vi "Generator.vi"(9 "Distance":dbl, 10 "Velocity Max":dbl, 11 "Acceleration Max":dbl) -> (2 "Velocity values":dbl[](array[numeric]), 3 "Timestamp":dbl[](array[numeric]) format="%.2f")   [LabVIEW 2023]
panel:
  out "area":sgl
  out "Time":sgl
  out "XY Graph":cluster{dbl[], dbl[]}(graph)
  out "Slope Change Point (seconds)":dbl
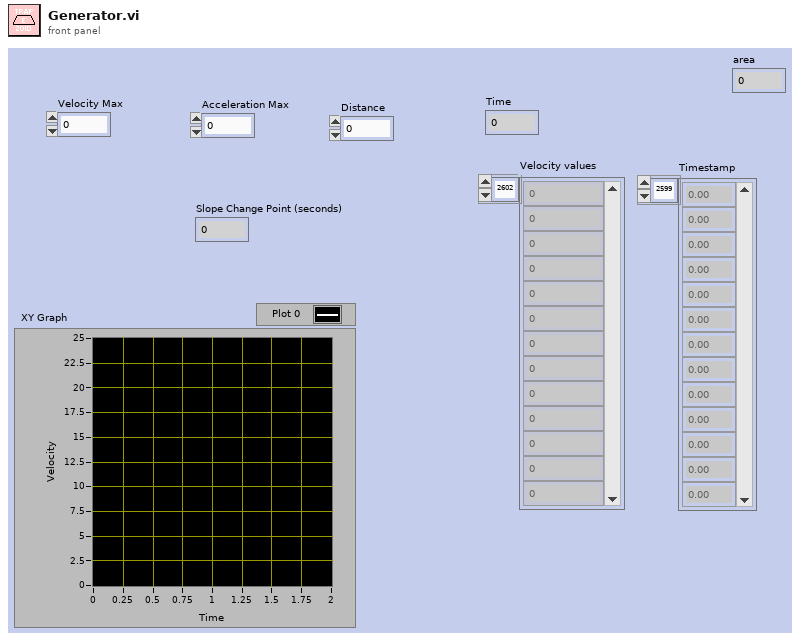
[diagram p1: front panel]
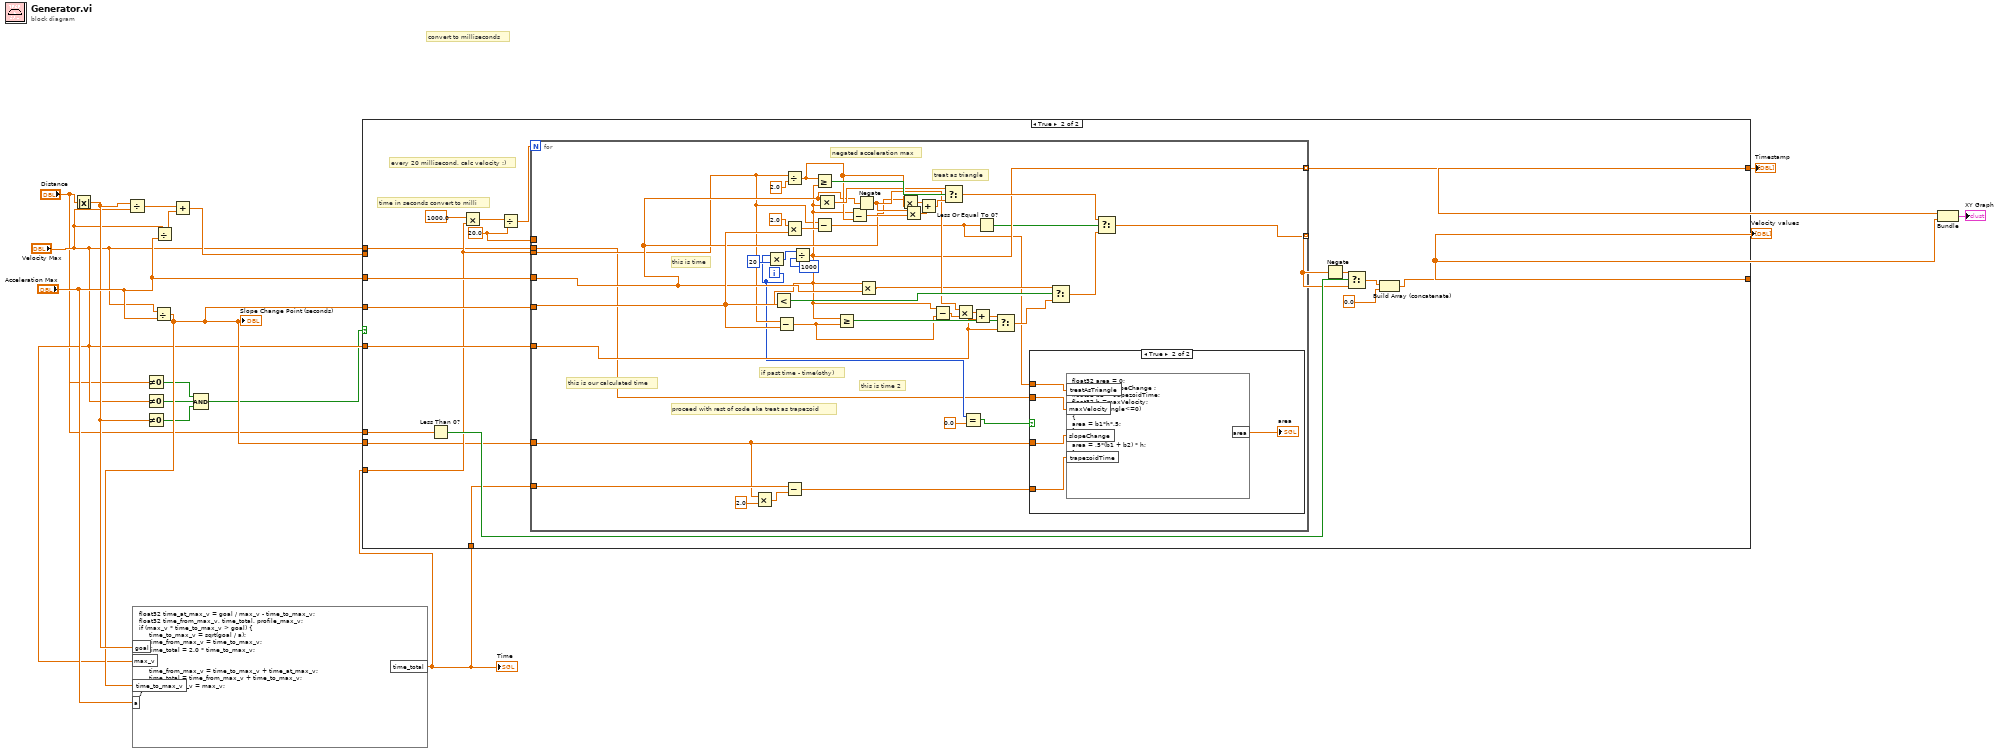
[diagram p0: block diagram]
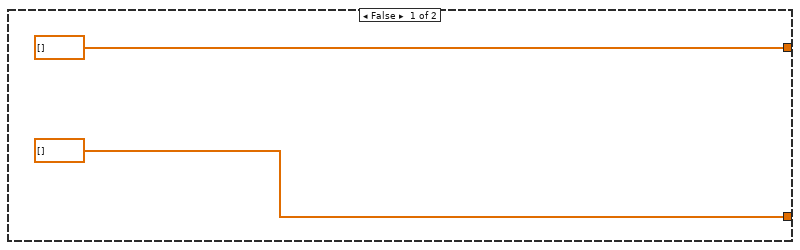
[diagram p2: hidden frame]
diagram:
  # "convert to milliseconds"
  n1 = Absolute Value(x="Distance") -> (abs(x)=w9:dbl)
  n2 = Divide(x=w9, y="Velocity Max") -> (x/y=w13:dbl)
  n3 = Not Equal To 0?(x="Distance") -> (x != 0?=w3:bool)
  n4 = Not Equal To 0?(x="Velocity Max") -> (x != 0?=w5:bool)
  n5 = Not Equal To 0?(x=w9) -> (x != 0?=w6:bool)
  n6 = Divide(x="Velocity Max", y="Acceleration Max") -> (x/y=w8:dbl)
  "Slope Change Point (seconds)" <- w8
  n7 = formula code="float32 time_at_max_v = goal / max_v - time_to_max_v;\nfloat32 time_from_max_v, time_total, profile_max_v;\nif (max_v * time_to_max_v > goal) {\n     time_to_max_v = sqrt(goal / a);\n     time_from_max_v = time_to_max_v;\n     time_total = 2.0 * time_to_max_v;\n}\nelse {\n     time_from_max_v = time_to_max_v + time_at_max_v;\n     time_total = time_from_max_v + time_to_max_v;\n     profile_max_v = max_v;\n}"("goal"=w9, "max_v"="Velocity Max", "time_to_max_v"=w8, "a"="Acceleration Max") -> ("time_total"=w7:sgl)
  "Time" <- w7
  n8 = Divide(x="Velocity Max", y="Acceleration Max") -> (x/y=w16:dbl)
  n9 = Add(x=w13, y=w16) -> (x+y=w14:dbl)
  n10 = Compound Arithmetic op=AND(w3, w5, w6) -> (w1:bool)
  n11 = case shown="True" w1 {
    tunnel: "Velocity Max" -> [_ w37]
    tunnel: w8 -> [_ w36]
    tunnel: [dbl[] [] w23] -> w15
    tunnel: w14 -> [_ _]
    tunnel: "Acceleration Max" -> [_ w34]
    tunnel: [dbl[] [] w24] -> w12
    tunnel: w7 -> [_ w22]
    tunnel: "Distance" -> [_ w29]
    tunnel: "Velocity Max" -> [_ w21]
    tunnel: w8 -> [_ w20]
    tunnel: w7 -> [_ w19]
    frame False {
    }
    frame True {
      w30 = 20.0 ("y")
      # "every 20 millisecond, calc velocity :)"
      # "time in seconds convert to milli"
      n12 = Less Than 0?(x=w29) -> (x < 0?=w32:bool)
      n13 = Multiply(x=1000.0, y=w22) -> (x*y=w35:dbl)
      n14 = Divide(x=w35, y=w30) -> (x/y=w27:dbl)
      n15 = for {
        N: w27 -> [_]
        tunnel: [w70] -> w31 mode=indexing
        tunnel: w34 -> [w60]
        tunnel: w37 -> [w52]
        tunnel: w36 -> [w69]
        tunnel: [w51] -> w23 mode=indexing
        tunnel: w30 -> [_]
        tunnel: w22 -> [w50]
        tunnel: w21 -> [w43]
        tunnel: w20 -> [w39]
        tunnel: w19 -> [w42]
        i -> [w45]
        # "this is our calculated time"
        # "this is time 2"
        # "this is time"
        # "negated acceleration max"
        # "if past time - time(othy)"
        # "treat as triangle"
        # "proceed with rest of code aka treat as trapezoid"
        n16 = Multiply(x=w39, y=2.0) -> (x*y=w41:dbl)
        n17 = Multiply(x=w45, y=20) -> (x*y=w57:i32)
        n18 = Subtract(x=w50, y=w69) -> (x-y=w58:dbl)
        n19 = Divide(x=w50, y=2.0) -> (x/y=w63:dbl)
        n20 = Multiply(x=2.0, y=w69) -> (x*y=w77:dbl)
        n21 = Subtract(x=w42, y=w41) -> (x-y=w38:dbl)
        n22 = Divide(x=w57, y=1000) -> (x/y=w51:dbl)
        n23 = Less?(x=w51, y=w69) -> (x < y?=w71:bool)
        n24 = Greater Or Equal?(x=w63, y=w51) -> (x >= y?=w75:bool)
        n25 = Subtract(x=w50, y=w77) -> (x-y=w44:dbl)
        n26 = Multiply(x=w60, y=w51) -> (x*y=w68:dbl)
        n27 = Greater Or Equal?(x=w51, y=w58) -> (x >= y?=w74:bool)
        n28 = Subtract(x=w51, y=w63) -> (x-y=w67:dbl)
        n29 = Negate(x=w60) -> (-x=w62:dbl)
        n30 = Multiply(x=w51, y=w60) -> (x*y=w55:dbl)
        n31 = Multiply(x=w60, y=w63) -> (x*y=w65:dbl)
        n32 = Multiply(x=w62, y=w67) -> (x*y=w66:dbl)
        n33 = Add(x=w65, y=w66) -> (x+y=w64:dbl)
        n34 = Subtract(x=w51, y=w58) -> (x-y=w53:dbl)
        n35 = Select(t=w68, s=w75, f=w64) -> (s? t:f=w59:dbl)
        n36 = Multiply(x=w62, y=w53) -> (x*y=w61:dbl)
        n37 = Equal?(x=w45, y=0.0) -> (x = y?=w47:bool)
        n38 = Add(x=w61, y=w52) -> (x+y=w54:dbl)
        n39 = Less Or Equal To 0?(x=w44) -> (x <= 0?=w48:bool)
        n40 = Select(t=w54, s=w74, f=w52) -> (s? t:f=w73:dbl)
        n41 = case shown="True" w47 {
          tunnel: w44 -> [_ w83]
          tunnel: w43 -> [_ w81]
          tunnel: w39 -> [_ w80]
          tunnel: w38 -> [_ w79]
          frame False {
          }
          frame True {
            n42 = formula code="float32 area = 0;\nfloat32 b1 =slopeChange ;\nfloat32 b2 = trapezoidTime;\nfloat32 h =maxVelocity; \nif(treatAsTriangle<=0)\n{\narea = b1*h*.5;\n}\nelse{\narea = .5*(b1 + b2) * h;\n}"("treatAsTriangle"=w83, "maxVelocity"=w81, "slopeChange"=w80, "trapezoidTime"=w79) -> ("area"=→"area":sgl)
          }
        }
        n43 = Select(t=w55, s=w71, f=w73) -> (s? t:f=w72:dbl)
        n44 = Select(t=w59, s=w48, f=w72) -> (s? t:f=w70:dbl)
      }
      n45 = Negate(x=w31) -> (-x=w33:dbl[])
      n46 = Select(t=w33, s=w32, f=w31) -> (s? t:f=w26:dbl[])
      n47 = Build Array (concatenate)(w26, 0.0) -> (w24:dbl[])
    }
  }
  "Velocity values" <- w12
  "Timestamp" <- w15
  n48 = Bundle(w15, w12) -> (→"XY Graph":cluster{dbl[], dbl[]})  [unwired: 1 in]
